vi "Speed angle to XYbvs.vi"(2 "Angle(deg)":dbl, 3 "dt(s)":dbl, 4 "Speed(km/h)":dbl) -> (0 "Y":dbl, 1 "x":dbl)   [LabVIEW 2022 SP3]
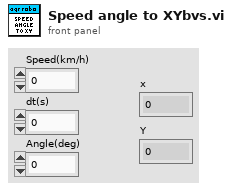
[diagram p1: front panel]
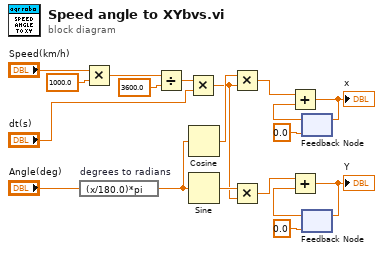
[diagram p0: block diagram]
diagram:
  n1 = expression code="(x/180.0)*pi" "degrees to radians"("Angle(deg)") -> (w15:dbl)
  n2 = Multiply(x="Speed(km/h)", y=1000.0) -> (x*y=w5:dbl)
  n3 = Divide(x=w5, y=3600.0) -> (x/y=w1:dbl)
  n4 = Multiply(x=w1, y="dt(s)") -> (x*y=w7:dbl)
  n5 = Cosine(x=w15) -> (cos(x)=w17:dbl)
  n6 = Sine(x=w15) -> (sin(x)=w16:dbl)
  n7 = Multiply(x=w17, y=w7) -> (x*y=w19:dbl)
  n8 = Multiply(x=w16, y=w7) -> (x*y=w18:dbl)
  n9 = feedback #1(0.0) -> (w8:dbl)
  n10 = Add(x=w19, y=w8) -> (x+y=w9:dbl)
  "x" <- w9
  n11 = feedback-in #1(w9) -> ()
  n12 = feedback #2(0.0) -> (w12:dbl)
  n13 = Add(x=w18, y=w12) -> (x+y=w13:dbl)
  "Y" <- w13
  n14 = feedback-in #2(w13) -> ()
